vi "Initialize Library.vi"(8 "error in (no error)":errorcluster) -> (0 "error out":errorcluster, 3 "Agilis out":T1)   [LabVIEW 2016, in "Drivers.lvlib" / "Agilis.lvlib"]
uses:
  Agilis.lvlib
  AgilisCmdLib Refnum.ctl
  C:/Users/Andy/Desktop/TraceGrabber/Drivers/Agilis/AgilisCmdLib.dll
  AgilisCmdLib.dll
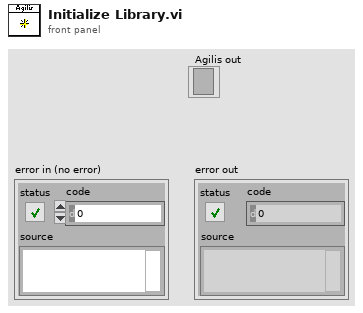
[diagram p1: front panel]
types:
  T1 = typedef "Drivers.lvlib/Agilis.lvlib/AgilisCmdLib Refnum.ctl" = refnum<k24>
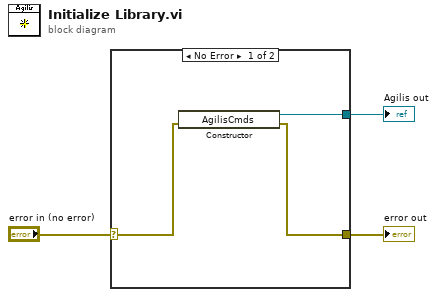
[diagram p0: block diagram]
diagram:
  n1 = case shown="No Error" "error in (no error)" {
    selector: "error in (no error)" -> [w4 w7]
    tunnel: [w6 _] -> w1
    tunnel: [w5 w7] -> w2
    frame No Error {
      n2 = constructor class="AgilisCmds"(error in=w4) -> (reference out=w6:refnum<k24>, error out=w5:errorcluster)  [unwired: 2 in, 1 out]
    }
    frame Error {
    }
  }
  "Agilis out" <- w1
  "error out" <- w2
